vi "System inquiry.vi"(8 "error in (no error)":errorcluster, 11 "VISA resource name":refnum<visa-resource-name>) -> (0 "error out":errorcluster, 1 "System":string, 2 "ID information":T1, 3 "VISA resource name out":refnum<visa-resource-name>)   [LabVIEW 2020, in "GPP.lvlib"]
uses:
  GPP.lvlib
  Function/VISA_COMMON.ctl
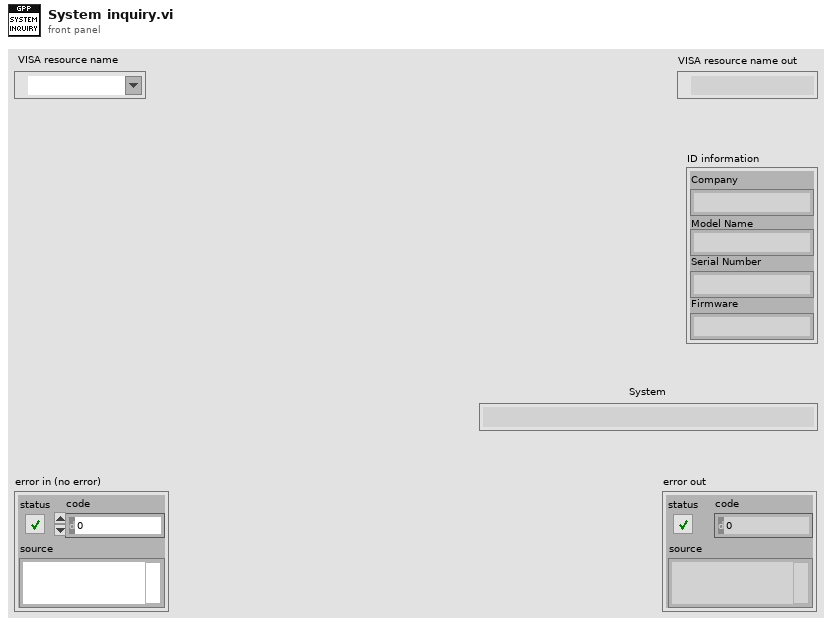
[diagram p1: front panel]
types:
  T1 = cluster{"Company":string, "Model Name":string, "Serial Number":string, "Firmware":string}
  T2 = typedef "GPP.lvlib/VISA_COMMON.ctl" = enum16{"Initial", "Write CMD", "Read Result", "Read History", "Close"}
  T3 = cluster{"[0]":string, "[1]":string, "[2]":string, "[3]":string}
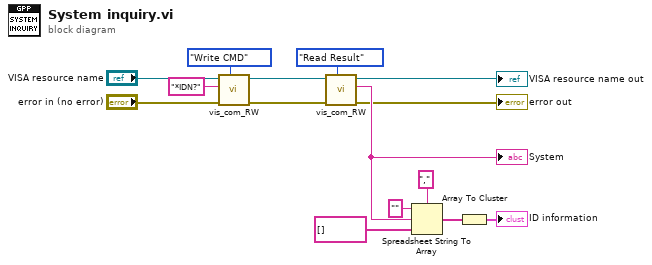
[diagram p0: block diagram]
diagram:
  n1 = call "vis_com_RW.vi"("Funciton"=VISA_COMMON."Write CMD", "error in (no error)"="error in (no error)", "CMD String"="*IDN?" ("ID Query"), "VISA resource in"="VISA resource name") -> ("error out"=w11:errorcluster, "VISA resource out"=w12:refnum<visa-resource-name>)  [unwired: 5 in, 1 out]
  n2 = call "vis_com_RW.vi"("Funciton"=VISA_COMMON."Read Result", "error in (no error)"=w11, "VISA resource in"=w12) -> ("error out"=→"error out":errorcluster, "Result"=w4:string, "VISA resource out"=→"VISA resource name out":refnum<visa-resource-name>)  [unwired: 6 in]
  "System" <- w4
  n3 = Spreadsheet String To Array(delimiter (Tab)=",", format string="", spreadsheet string=w4, array type (2D Dbl)=string[] []) -> (array=w6:string[])
  n4 = Array To Cluster(array=w6) -> (cluster=→"ID information":T3)
